vi "Get last state.vi"(0 "Datalog directory path":path) -> (2 "Plant State":T2=1 items=["OFF"], 3 "Plant Mode of Operation":T1=enum."Automatic Operation")   [LabVIEW 2015]
uses:
  Plant state.ctl
  Plant mode.ctl
  <vilib>/Utility/file.llb/Read From Spreadsheet File (DBL).vi
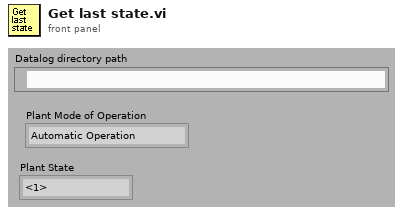
[diagram p1: front panel]
types:
  T1 = typedef "Plant mode.ctl" = enum16{"Manual Locked in State", "Automatic Operation"}
  T2 = typedef "Plant state.ctl" = u16
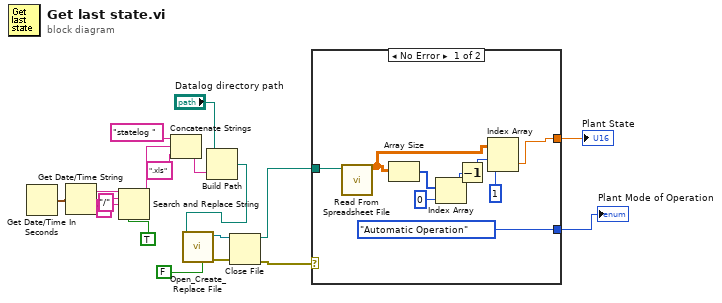
[diagram p0: block diagram]
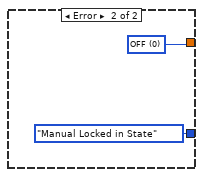
[diagram p2: hidden frame]
diagram:
  n1 = Get Date/Time In Seconds() -> (seconds since 1Jan1904=w9:timestamp)
  n2 = Get Date/Time String(seconds (now)=w9) -> (date string=w11:string)  [unwired: 2 in, 1 out]
  n3 = Search and Replace String(replace all?=TRUE ("replace all? (F)"), input string=w11, search string="/", replace string="-" ("replace string (\"\")")) -> (result string=w14:string)  [unwired: 4 in, 3 out]
  n4 = Concatenate Strings("statelog " ("string"), w14, ".xls" ("string")) -> (w13:string)
  n5 = Build Path(base path="Datalog directory path", name or relative path=w13) -> (appended path=w4:path)
  n6 = call <vilib>:"Open_Create_Replace File.vi"("advisory dialog? (display:T)"=FALSE, "file path"=w4) -> ("error out"=w6:errorcluster, "refnum"=w5:refnum<file>)  [unwired: 6 in, 2 out]
  n7 = Close File(refnum=w5, error in=w6) -> (path=w3:path, error out=w2:errorcluster)
  n8 = case shown="No Error" w2 {
    tunnel: [w27 w28] -> w10
    tunnel: [Plant_mode."Automatic Operation" ("Plant Mode of Operation") Plant_mode."Manual Locked in State" ("Plant Mode of Operation")] -> w8
    tunnel: w3 -> [w25 _]
    frame No Error {
      n9 = call-poly <vilib>:"Read From Spreadsheet File.vi"("file path (dialog if empty)"=w25) -> ("all rows"=w24:dbl[][])  [unwired: 6 in, 4 out]
      n10 = Array Size(array=w24) -> (size(s)=w23:i32[])
      n11 = Index Array(array=w23, index=0) -> (element=w21:i32)
      n12 = Decrement(x=w21) -> (x-1=w20:i32)
      n13 = Index Array(array=w24, index (row)=w20, index (col)=1 ("disabled index (col)")) -> (element=w27:dbl)
    }
    frame Error {
      w28 = T2 0 items=["OFF"] ("Plant State")
    }
  }
  "Plant State" <- w10
  "Plant Mode of Operation" <- w8
